vi "Second1.vi"() -> ()   [LabVIEW 2020]
uses:
  First1Second1glb.vi
panel:
  out "Waveform Chart":i32(graph)
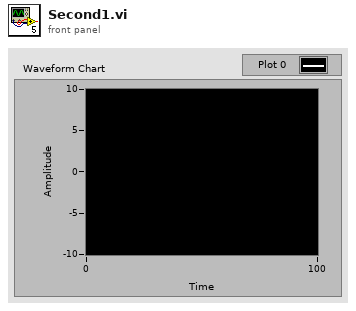
[diagram p1: front panel]
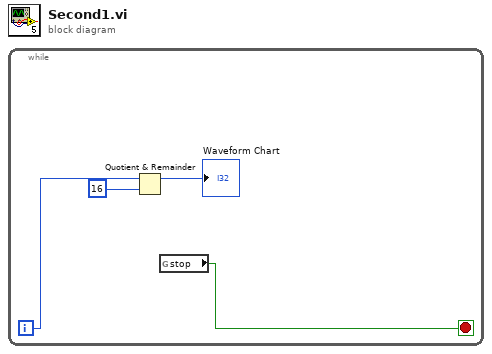
[diagram p0: block diagram]
diagram:
  n1 = while {
    i -> [w4]
    stop <- w1 stop-if-true
    n2 = Quotient & Remainder(x=w4, y=16) -> (x-y*floor(x/y)=→"Waveform Chart":i32)  [unwired: 1 out]
    n3 = global read "First1Second1glb.vi" "stop"() -> (w1:bool)
  }
